vi "Gimbal 2.vi"(2 "frequency (periods/tick)":fxp<+,32,0>, 5 "PITCH 2":fxp<+,32,0>, 9 "ROLL2":fxp<+,32,0>, 11 "YAW 2":fxp<+,32,0>) -> (4 "DIO 10":bool, 6 "DIO 11":bool, 15 "DIO 12":bool)   [LabVIEW 2015]
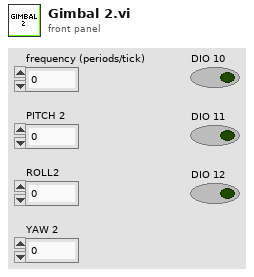
[diagram p1: front panel]
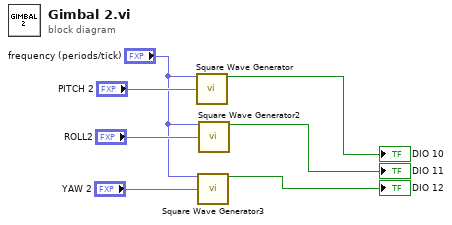
[diagram p0: block diagram]
diagram:
  n1 = call "Square Wave Generator"("frequency (periods/tick)"="frequency (periods/tick)", "duty cycle (periods)"="PITCH 2") -> ("square wave out"=→"DIO 10":bool)  [unwired: 13 in]
  n2 = call "Square Wave Generator3"("frequency (periods/tick)"="frequency (periods/tick)", "duty cycle (periods)"="YAW 2") -> ("square wave out"=→"DIO 12":bool)  [unwired: 13 in]
  n3 = call "Square Wave Generator2"("frequency (periods/tick)"="frequency (periods/tick)", "duty cycle (periods)"="ROLL2") -> ("square wave out"=→"DIO 11":bool)  [unwired: 13 in]
